vi "Master Reference Not Closed--error.vi"() -> (0 "error out":errorcluster)   [LabVIEW 2024, in "Clon.lvlib"]
doc: "Outputs an error cluster containing a custom error code indicating the module cannot be run as singleton because it was previously run as cloneable and the master reference is still open.\n_____\nBased on DQMH Dev Tools: Project Template 7.1.0.1503."
uses:
  Clon.lvlib
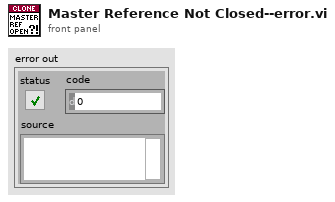
[diagram p1: front panel]
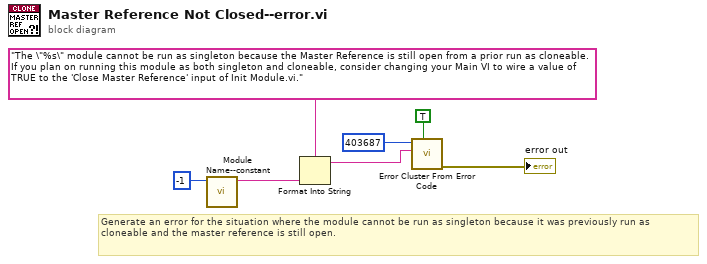
[diagram p0: block diagram]
diagram:
  # "Generate an error for the situation where the module cannot be run as singleton because it was previously run as cloneable and the master reference is still open."
  n1 = call "Module Name--constant.vi"("Module ID"=-1) -> ("Module Name"=w6:string)  [unwired: 10 in]
  n2 = Format Into String(format string="The \"%s\" module cannot be run as singleton because the Master Reference is still open from a prior run as cloneable. If you plan on running this module as both singleton and cloneable, consider changing your Main VI to wire a value of TRUE to the 'Close Master Reference' input of Init Module.vi.", w6) -> (resulting string=w4:string)  [unwired: 2 in, 1 out]
  n3 = call <vilib>:"Error Cluster From Error Code.vi"("show call chain? (False)"=TRUE, "error message (\"\")"=w4, "error code (0)"=403687) -> ("error out"=→"error out":errorcluster)  [unwired: 6 in]
